vi "Dynamic Scaffold.vi"(11 "Object":T2) -> ()   [LabVIEW 2018, in "LVClassByRef.lvlib"]
uses:
  <resource>/Framework/Providers/LVClassByRef/LVClassByRef.lvlib
  <resource>/Framework/Providers/API/ItemRef.ctl
  <resource>/Framework/Providers/LVClassByRef/Scaffold Steps.ctl
  <resource>/Framework/Providers/LVClassByRef/Static Build Ctor Scripting.vi
  <resource>/Framework/Providers/LVClassByRef/Build Cleanup Scripting.vi
  <resource>/Framework/Providers/LVClassByRef/Cleanup Template.vit
panel:
  out "Status":string
  out "error in (no error)":errorcluster
  out "State":T1
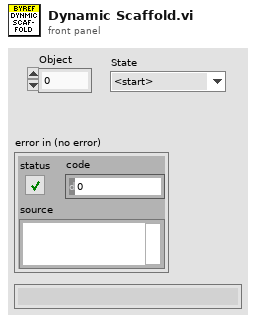
[diagram p1: front panel]
types:
  T1 = typedef "LVClassByRef.lvlib/Scaffold Steps.ctl" = enum16{"<start>", "Files Folder", "Private Folder", "Protected Folder", "Community Folder", "Properties Folder", "Public Folder", "Priv DataTypes Folder", "Pub DataTypes Folder", "RefData Ctl", "Ctor VI", "Cleanup VI", "<done>"}
  T2 = typedef "ItemRef.ctl" = u64
  T3 = typedef "LVClassByRef.lvlib/Scaffold Project Refs.ctl" = cluster{"Class":refnum<vi>, "Class Data":refnum<vi>, "Files VF":refnum<vi>, "Private VF":refnum<vi>, "Protected VF":refnum<vi>, "Community VF":refnum<vi>, "Public VF":refnum<vi>, "Priv_DataTypes VF":refnum<vi>, "Pub_DataTypes VF":refnum<vi>, "RefData Ctl":refnum<vi>, "Ctor VI":refnum<vi>, "Cleanup VI":refnum<vi>, "Properties VF":refnum<vi>}
  T4 = enum32{"invalid scope", "public", "private", "protected", "community"}
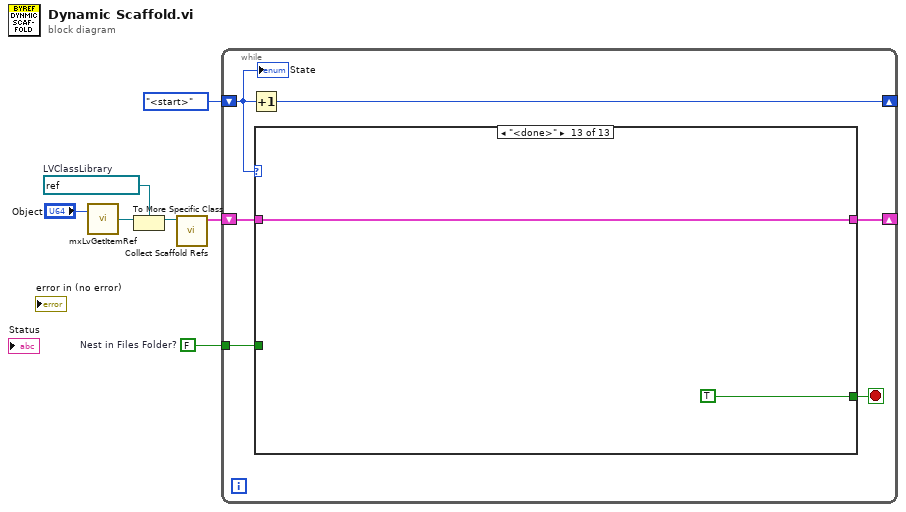
[diagram p0: block diagram]
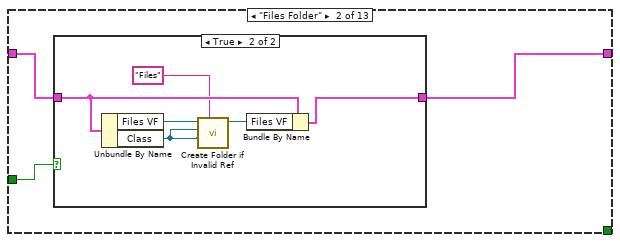
[diagram p3: hidden frame]
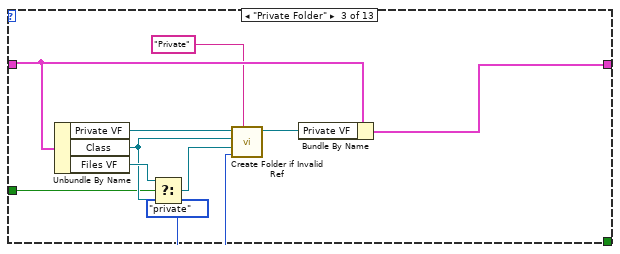
[diagram p5: hidden frame]
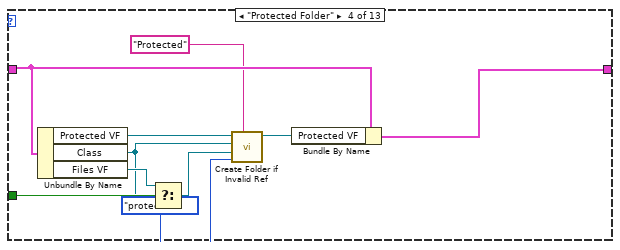
[diagram p6: hidden frame]
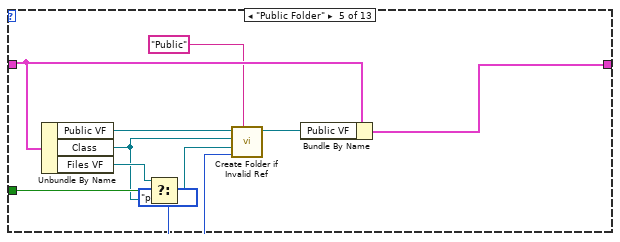
[diagram p7: hidden frame]
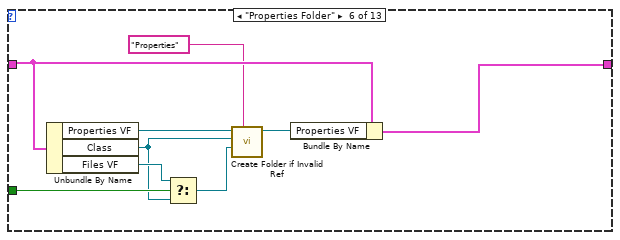
[diagram p8: hidden frame]
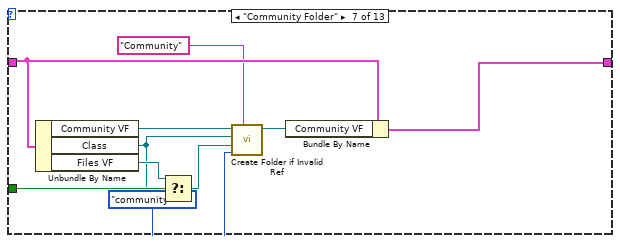
[diagram p9: hidden frame]
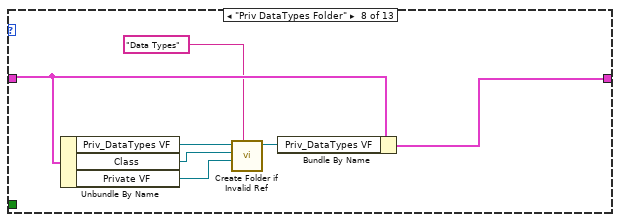
[diagram p10: hidden frame]
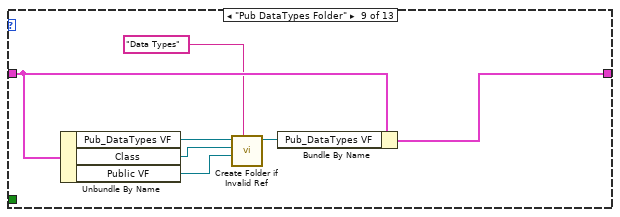
[diagram p11: hidden frame]
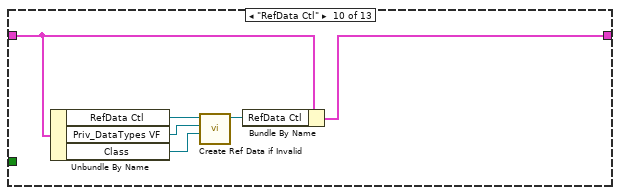
[diagram p12: hidden frame]
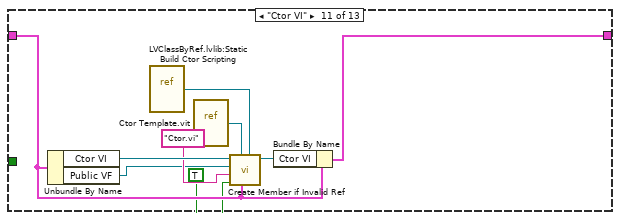
[diagram p13: hidden frame]
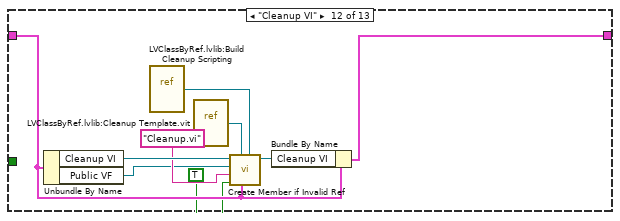
[diagram p14: hidden frame]
diagram:
  w1 = FALSE  # Nest in Files Folder?
  w4 = refnum<vi> refnum  # LVClassLibrary
  n1 = call <resource>:"mxLvGetItemRef.vi"("Item"="Object") -> ("Item Refnum"=w5:refnum<vi>)  [unwired: 1 in, 2 out]
  n2 = To More Specific Class(target class=w4, reference=w5) -> (specific class reference=w3:refnum<vi>)  [unwired: 1 in, 1 out]
  n3 = call <resource>:"Collect Scaffold Refs.vi"("Class Item"=w3) -> ("Scaffold Project Refs"=w2:T3)  [unwired: 10 in]
  n4 = while {
    shift-right: [w10] -> _
    shift-left: w2 -> [w11]
    shift-right: [w13] -> _
    shift-left: Scaffold_Steps."<start>" ("Scaffold Steps") -> [w12]
    tunnel: w1 -> [w8]
    stop <- w9 stop-if-true
    n5 = Increment(x=w12) -> (x+1=w13:T1)
    n6 = case shown="\"<done>\"" w12 {
      tunnel: w11 -> [w14 w17 w32 w42 w52 w61 w71 w78 w85 w93 w98 w107 w112]
      tunnel: [w14 w16 w31 w41 w51 w60 w70 w77 w84 w89 w96 w105 w112] -> w10
      tunnel: [_ _ _ _ _ _ _ _ _ _ _ _ TRUE] -> w9
      tunnel: w8 -> [_ w15 w26 w38 w48 w57 w67 _ _ _ _ _ _]
      frame "<start>" {
      }
      frame "Files Folder" {
        n7 = case shown="True" w15 {
          tunnel: w17 -> [w18 w23]
          tunnel: [w18 w21] -> w16
          frame False {
          }
          frame True {
            n8 = Unbundle By Name(w23) -> ("Files VF"=w24:refnum<vi>, "Class"=w20:refnum<vi>)
            n9 = call <resource>:"Create Folder if Invalid Ref.vi"("Name"="Files", "Parent"=w20, "Library"=w20, "Folder Ref In"=w24) -> ("Folder Ref"=w22:refnum<vi>)  [unwired: 7 in]
            n10 = Bundle By Name(cluster=w23, "Files VF"=w22) -> (w21:T3)
          }
        }
      }
      frame "Private Folder" {
        n11 = Unbundle By Name(w32) -> ("Private VF"=w34:refnum<vi>, "Class"=w27:refnum<vi>, "Files VF"=w28:refnum<vi>)
        n12 = Select(t=w28, s=w26, f=w27) -> (s? t:f=w25:refnum<vi>)
        n13 = call <resource>:"Create Folder if Invalid Ref.vi"("Name"="Private", "Access Scope (none)"=T4."private", "Parent"=w25, "Library"=w27, "Folder Ref In"=w34) -> ("Folder Ref"=w33:refnum<vi>)  [unwired: 6 in]
        n14 = Bundle By Name(cluster=w32, "Private VF"=w33) -> (w31:T3)
      }
      frame "Protected Folder" {
        n15 = Unbundle By Name(w42) -> ("Protected VF"=w44:refnum<vi>, "Class"=w36:refnum<vi>, "Files VF"=w37:refnum<vi>)
        n16 = Select(t=w37, s=w38, f=w36) -> (s? t:f=w35:refnum<vi>)
        n17 = call <resource>:"Create Folder if Invalid Ref.vi"("Name"="Protected", "Access Scope (none)"=T4."protected", "Parent"=w35, "Library"=w36, "Folder Ref In"=w44) -> ("Folder Ref"=w43:refnum<vi>)  [unwired: 6 in]
        n18 = Bundle By Name(cluster=w42, "Protected VF"=w43) -> (w41:T3)
      }
      frame "Public Folder" {
        n19 = Unbundle By Name(w52) -> ("Public VF"=w54:refnum<vi>, "Class"=w46:refnum<vi>, "Files VF"=w47:refnum<vi>)
        n20 = Select(t=w47, s=w48, f=w46) -> (s? t:f=w45:refnum<vi>)
        n21 = call <resource>:"Create Folder if Invalid Ref.vi"("Name"="Public", "Access Scope (none)"=T4."public", "Parent"=w45, "Library"=w46, "Folder Ref In"=w54) -> ("Folder Ref"=w53:refnum<vi>)  [unwired: 6 in]
        n22 = Bundle By Name(cluster=w52, "Public VF"=w53) -> (w51:T3)
      }
      frame "Properties Folder" {
        n23 = Unbundle By Name(w61) -> ("Properties VF"=w63:refnum<vi>, "Class"=w56:refnum<vi>, "Files VF"=w58:refnum<vi>)
        n24 = Select(t=w58, s=w57, f=w56) -> (s? t:f=w55:refnum<vi>)
        n25 = call <resource>:"Create Folder if Invalid Ref.vi"("Name"="Properties", "Parent"=w55, "Library"=w56, "Folder Ref In"=w63) -> ("Folder Ref"=w62:refnum<vi>)  [unwired: 7 in]
        n26 = Bundle By Name(cluster=w61, "Properties VF"=w62) -> (w60:T3)
      }
      frame "Community Folder" {
        n27 = Unbundle By Name(w71) -> ("Community VF"=w73:refnum<vi>, "Class"=w65:refnum<vi>, "Files VF"=w66:refnum<vi>)
        n28 = Select(t=w66, s=w67, f=w65) -> (s? t:f=w64:refnum<vi>)
        n29 = call <resource>:"Create Folder if Invalid Ref.vi"("Name"="Community", "Access Scope (none)"=T4."community", "Parent"=w64, "Library"=w65, "Folder Ref In"=w73) -> ("Folder Ref"=w72:refnum<vi>)  [unwired: 6 in]
        n30 = Bundle By Name(cluster=w71, "Community VF"=w72) -> (w70:T3)
      }
      frame "Priv DataTypes Folder" {
        n31 = Unbundle By Name(w78) -> ("Priv_DataTypes VF"=w80:refnum<vi>, "Class"=w75:refnum<vi>, "Private VF"=w74:refnum<vi>)
        n32 = call <resource>:"Create Folder if Invalid Ref.vi"("Name"="Data Types", "Parent"=w74, "Library"=w75, "Folder Ref In"=w80) -> ("Folder Ref"=w79:refnum<vi>)  [unwired: 7 in]
        n33 = Bundle By Name(cluster=w78, "Priv_DataTypes VF"=w79) -> (w77:T3)
      }
      frame "Pub DataTypes Folder" {
        n34 = Unbundle By Name(w85) -> ("Pub_DataTypes VF"=w87:refnum<vi>, "Class"=w82:refnum<vi>, "Public VF"=w81:refnum<vi>)
        n35 = call <resource>:"Create Folder if Invalid Ref.vi"("Name"="Data Types", "Parent"=w81, "Library"=w82, "Folder Ref In"=w87) -> ("Folder Ref"=w86:refnum<vi>)  [unwired: 7 in]
        n36 = Bundle By Name(cluster=w85, "Pub_DataTypes VF"=w86) -> (w84:T3)
      }
      frame "RefData Ctl" {
        n37 = Unbundle By Name(w93) -> ("RefData Ctl"=w92:refnum<vi>, "Priv_DataTypes VF"=w91:refnum<vi>, "Class"=w90:refnum<vi>)
        n38 = call <resource>:"Create Ref Data if Invalid.vi"("Class"=w90, "Folder"=w91, "Ref Data In"=w92) -> ("Ref Data"=w88:refnum<vi>)  [unwired: 7 in, 1 out]
        n39 = Bundle By Name(cluster=w93, "RefData Ctl"=w88) -> (w89:T3)
      }
      frame "Ctor VI" {
        n40 = Unbundle By Name(w98) -> ("Ctor VI"=w100:refnum<vi>, "Public VF"=w94:refnum<vi>)
        n41 = vi-ref "LVClassByRef.lvlib:Static Build Ctor Scripting.vi"() -> (w102:refnum<vi>)
        n42 = vi-ref <resource>:"Ctor Template.vit"() -> (w101:refnum<vi>)
        n43 = call <resource>:"Create Member if Invalid Ref.vi"("Additional Scripting Ref"=w102, "Scaffold Project Refs"=w98, "Member Template"=w101, "Dynamic?"=TRUE, "Member Name"="Ctor.vi", "Parent"=w94, "Member In"=w100) -> ("Member ProjectItem"=w97:refnum<vi>)  [unwired: 4 in]
        n44 = Bundle By Name(cluster=w98, "Ctor VI"=w97) -> (w96:T3)
      }
      frame "Cleanup VI" {
        n45 = Unbundle By Name(w107) -> ("Cleanup VI"=w109:refnum<vi>, "Public VF"=w103:refnum<vi>)
        n46 = vi-ref "LVClassByRef.lvlib:Build Cleanup Scripting.vi"() -> (w111:refnum<vi>)
        n47 = vi-ref "LVClassByRef.lvlib:Cleanup Template.vit"() -> (w110:refnum<vi>)
        n48 = call <resource>:"Create Member if Invalid Ref.vi"("Additional Scripting Ref"=w111, "Scaffold Project Refs"=w107, "Member Template"=w110, "Dynamic?"=TRUE, "Member Name"="Cleanup.vi", "Parent"=w103, "Member In"=w109) -> ("Member ProjectItem"=w106:refnum<vi>)  [unwired: 4 in]
        n49 = Bundle By Name(cluster=w107, "Cleanup VI"=w106) -> (w105:T3)
      }
      frame "<done>" {
      }
    }
    "State" <- w12
  }
